vi "Run.vi"(8 "error in (no error)":errorcluster caption="entrée d'erreur (pas d'erreur)", 11 "Olivetti_faces.lvclass":refnum<class "Olivetti_faces.lvclass">) -> (0 "error out":errorcluster caption="sortie d'erreur", 2 "Data":T1, 3 "Olivetti_faces.lvclass":refnum<class "Olivetti_faces.lvclass">)   [LabVIEW 2020, in "Olivetti_faces.lvclass"]
doc: "Returns :\n\n- data : ndarray, shape (400, 64, 64)\nEach row is a face image corresponding to one of the 40 subjects of the dataset.\n\n- target : ndarray, shape (400,)\nLabels associated to each face image. Those labels are ranging from 0-39 and correspond to the Subject IDs."
uses:
  Olivetti_faces.lvclass
  Olivetti_faces.lvclass/Olivetti_faces.ctl
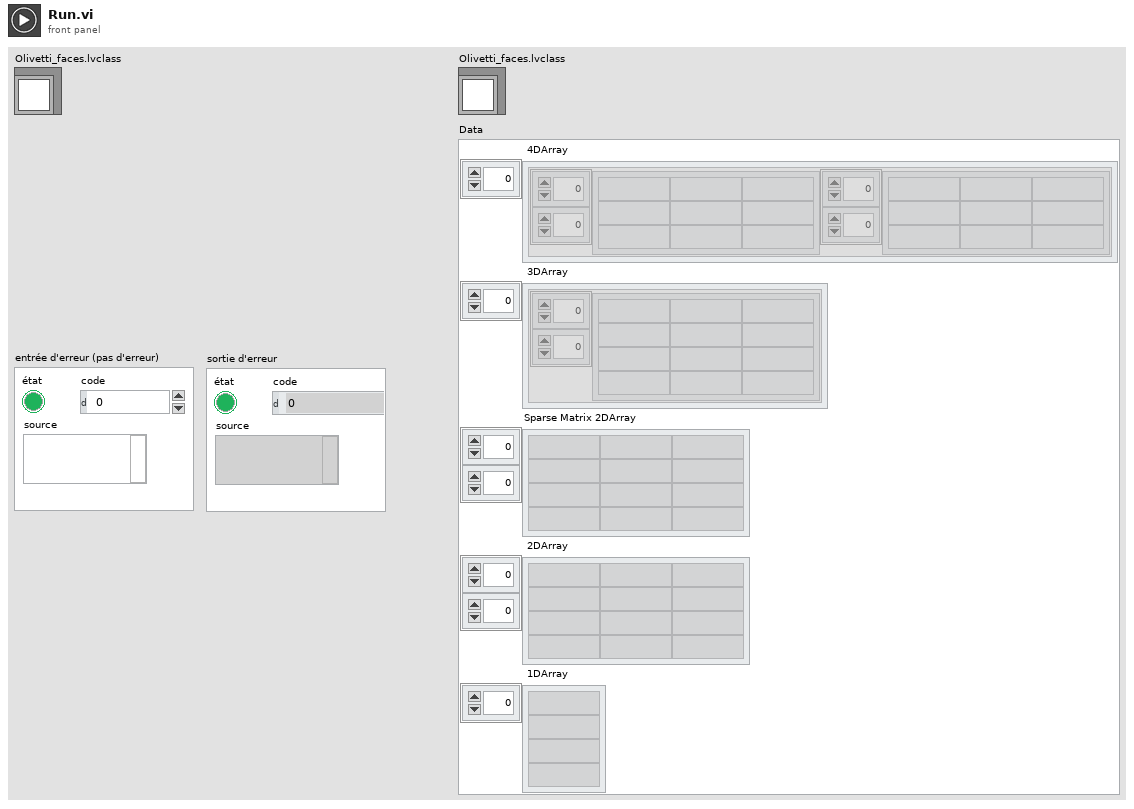
[diagram p1: front panel]
types:
  T1 = cluster{" 4DArray":cluster{"1":string[][], "2":string[][]}[], " 3DArray":cluster{"Tableau":string[][]}[], "Sparse Matrix 2DArray":string[][], " 2DArray":string[][], " 1DArray":string[]}
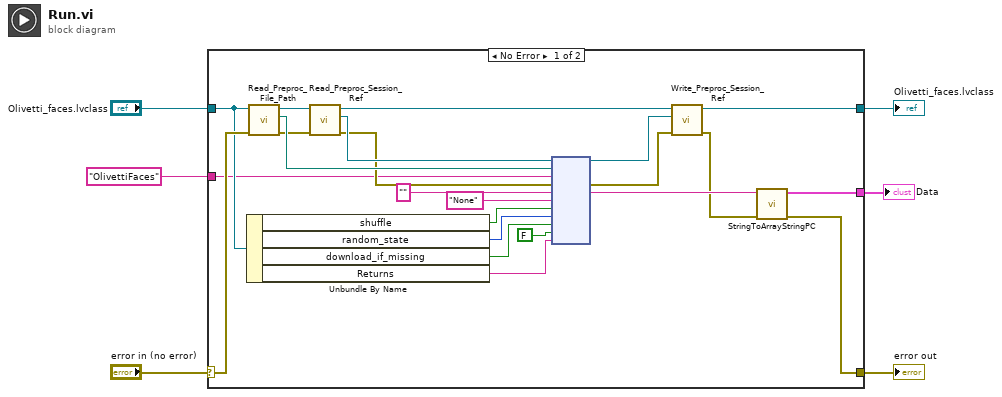
[diagram p0: block diagram]
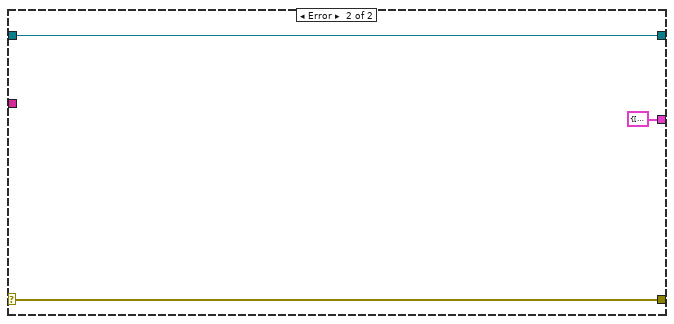
[diagram p2: hidden frame]
diagram:
  n1 = case shown="No Error" "error in (no error)" {
    selector: "error in (no error)" -> [w22 w32]
    tunnel: [w8 w32] -> w5
    tunnel: [w11 w31] -> w3
    tunnel: "Olivetti_faces.lvclass" -> [w21 w31]
    tunnel: "OlivettiFaces" -> [w20 _]
    tunnel: [w7 T1 {" 4DArray"=[], " 3DArray"=[], "Sparse Matrix 2DArray"=[], " 2DArray"=[], " 1DArray"=[]} ("Data")] -> w1
    frame No Error {
      n2 = Unbundle By Name(w21) -> ("shuffle"=w19:bool, "random_state"=w18:i32, "download_if_missing"=w16:bool, "Returns"=w12:string)
      n3 = call-dynamic "Read_Preproc_File_Path.vi"("error in (no error)"=w22, "Python in"=w21) -> ("error out"=w24:errorcluster, "File_Path"=w27:path, "Python out"=w29:refnum<class "Olivetti_faces.lvclass">)  [unwired: 7 in]
      n4 = call-dynamic "Read_Preproc_Session_Ref.vi"("error in (no error)"=w24, "Python in"=w29) -> ("error out"=w25:errorcluster, "Session_ref"=w26:refnum<k35>, "Python out"=w28:refnum<class "Olivetti_faces.lvclass">)  [unwired: 7 in]
      n5 = node(w26, w27, w20, w25, "", "None", w19, w18, w16, FALSE, w12) -> (w14:refnum<k35>, w13:errorcluster, w10:string)  [unwired: 6 in, 2 out]
      n6 = call-dynamic "Write_Preproc_Session_Ref.vi"("error in (no error)"=w13, "Session_ref"=w14, "Python in"=w28) -> ("error out"=w9:errorcluster, "Python out"=w11:refnum<class "Olivetti_faces.lvclass">)  [unwired: 7 in]
      n7 = call "StringToArrayStringPC.vi"("sortie d'erreur"=w9, "Return value"=w10) -> ("sortie d'erreur"=w8:errorcluster, "Data"=w7:T1)  [unwired: 8 in]
    }
    frame Error {
    }
  }
  "error out" <- w5
  "Olivetti_faces.lvclass" <- w3
  "Data" <- w1
